vi "asset.create_free.vi"(8 "error in":errorcluster, 11 "AssetCreateStaging in":refnum<class "AssetCreateStaging.lvclass">) -> (0 "error out":errorcluster)   [LabVIEW 2020, in "AssetCreateStaging.lvclass"]
doc: "Releases the handle and its associated resources."
uses:
  AssetCreateStaging.lvclass
  AssetCreateStaging.lvclass/AssetCreateStaging.ctl
  client.lvlib
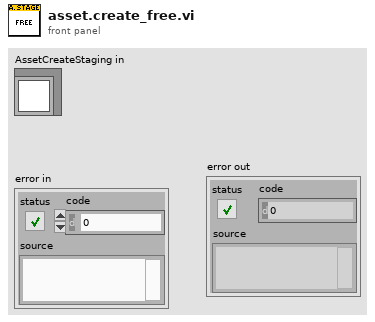
[diagram p1: front panel]
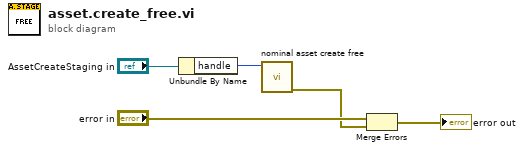
[diagram p0: block diagram]
diagram:
  n1 = Unbundle By Name("AssetCreateStaging in") -> ("handle"=w5:i32)
  n2 = call "nominal asset create free.vi"("staging"=w5) -> ("error out"=w2:errorcluster)  [unwired: 9 in, 1 out]
  n3 = Merge Errors("error in", w2) -> (→"error out":errorcluster)
